vi "Auto Indexer.vi"(8 "error in (no error)":errorcluster, 10 "T=Reverse":bool, 11 "T=Forward":bool) -> (0 "error out":errorcluster)   [LabVIEW 2014]
uses:
  <vilib>/Rock Robotics/WPI/Relay/WPI_RelayValue.ctl
  Global Variables/Global Variables.vi
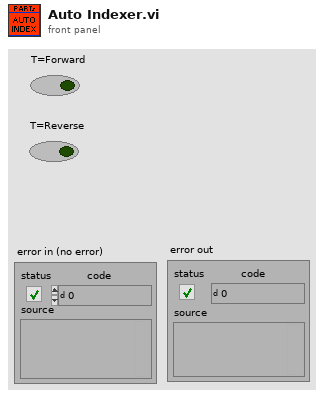
[diagram p1: front panel]
types:
  T1 = typedef "WPI_RelayValue.ctl" = enum16{"Off", "On", "Forward", "Reverse"}
  T2 = typedef "WPI_RelayDevRef.ctl" = cluster{"DevStatus":errorcluster, "Relay Channel":T3, "Controller":T4, "Relay Direction":T5}
  T3 = typedef "FPGA_DIORelayChannel.ctl" = enum8{"Relay 0", "Relay 1", "Relay 2", "Relay 3", "Invalid"}
  T4 = typedef "FPGA_TypedefDigitalModule.ctl" = enum16{"Controller 1"}
  T5 = typedef "WPI_RelayDirection.ctl" = enum16{"Both directions", "Forward only", "Reverse only"}
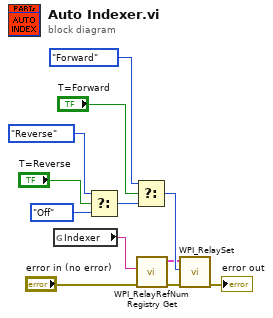
[diagram p0: block diagram]
diagram:
  n1 = global read "Global Variables.vi" "Indexer"() -> (w5:string)
  n2 = Select(t=WPI_RelayValue."Reverse" ("RelayValue"), s="T=Reverse", f=WPI_RelayValue."Off" ("RelayValue")) -> (s? t:f=w10:T1)
  n3 = Select(t=WPI_RelayValue."Forward" ("RelayValue"), s="T=Forward", f=w10) -> (s? t:f=w9:T1)
  n4 = call <vilib>:"WPI_RelayRefNum Registry Get.vi"("error in (no error)"="error in (no error)", "refnum name"=w5) -> ("error out"=w7:errorcluster, "RelayDevRef"=w6:T2)  [unwired: 8 in]
  n5 = call <vilib>:"WPI_RelaySet.vi"("error in (no error)"=w7, "RelayValue"=w9, "RelayDevRef"=w6) -> ("error out"=→"error out":errorcluster)  [unwired: 7 in, 1 out]
